vi "SIM Adams resample BDs.vi"(3 "Adams data":T1, 4 "current stepSize":dbl, 5 "new stepSize":dbl) -> (0 "Adams data out":T1)   [LabVIEW 2020]
uses:
  SIM Adams data.ctl
  SIM Adams stages.ctl
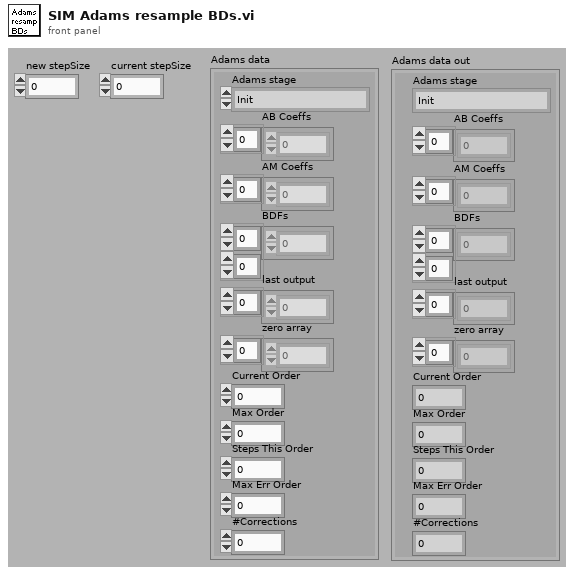
[diagram p1: front panel]
types:
  T1 = typedef "SIM Adams data.ctl" = cluster{"Adams stage":T2, "AB Coeffs":dbl[], "AM Coeffs":dbl[], "BDFs":dbl[][], "last output":dbl[], "zero array":dbl[], "Current Order":i32, "Max Order":i32, "Steps This Order":i32, "Max Err Order":i32, "#Corrections":i32}
  T2 = typedef "SIM Adams stages.ctl" = enum16{"Init", "Predict", "Correct", "Eval Error", "Choose StepSize", "Reset BDFs"}
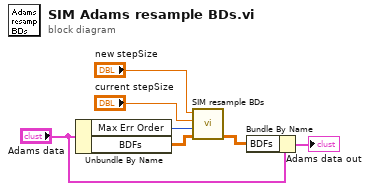
[diagram p0: block diagram]
diagram:
  n1 = Unbundle By Name("Adams data") -> ("Max Err Order"=w7:i32, "BDFs"=w1:dbl[][])
  n2 = call "SIM resample BDs.vi"("Backward differences"=w1, "interp poly order"=w7, "current timestep"="current stepSize", "new timestep"="new stepSize") -> ("New Backward differences"=w3:dbl[][])  [unwired: 7 out]
  n3 = Bundle By Name(cluster="Adams data", "BDFs"=w3) -> (→"Adams data out":T1)
